vi "FeedbackDecode.vi"() -> ()   [LabVIEW 2020] (continued)
        n285 = call "FeedbackDecode_PlotHeatmap.vi"("Range"=w3314, "GridIntensity"=w3326, "Instance"=0, "Mode"=w3331) -> ("Pic"=w3317:picture)  [unwired: 2 in, 1 out]
        n286 = call "FeedbackDecode_PlotHeatmap.vi"("Range"=w3314, "GridIntensity"=w3325, "Instance"=1, "Mode"=w3331) -> ("Pic"=w3316:picture)  [unwired: 2 in, 1 out]
        n287 = call "FeedbackDecode_PlotHeatmap.vi"("Range"=w3314, "GridIntensity"=w3318, "Instance"=2, "Mode"=w3331) -> ("Pic"=w3315:picture)  [unwired: 2 in, 1 out]
        n288 = local write "MedianHM"(w3317) -> ()
        n289 = local write "UlnarHM"(w3316) -> ()
        n290 = local write "EMGHM"(w3315) -> ()
        n291 = for {
          tunnel: w3258 -> [w3411] mode=indexing
          tunnel: [w3410] -> w3260 mode=indexing
          tunnel: w3259 -> [w3407]
          tunnel: w3257 -> [w3409] mode=indexing
          tunnel: [w3406] -> w3256 mode=indexing
          n292 = Build Array(w3411) -> (w3412:dbl[])
          n293 = Build Array(w3409) -> (w3408:dbl[])
          n294 = Bundle By Name("Y"=w3412, "t0"=w3407) -> (w3410:waveform(dbl))  [unwired: 1 in]
          n295 = Bundle By Name("Y"=w3408, "t0"=w3407) -> (w3406:waveform(dbl))  [unwired: 1 in]
        }
        "TASKA Pressure" <- w3260
        "TASKA IR" <- w3256
        n296 = global read "FeedbackDecode_Globals.vi" "FD_PupilClust"() -> (→"PupilClust":T11)
        n297 = case shown="True" w3263 {
          frame False {
          }
          frame True {
            n298 = call <vilib>:"Play Sound File.vi"("path"=path "C:/Windows/Media/Windows Critical Stop.wav") -> ()  [unwired: 9 in, 2 out]
          }
        }
        n299 = local read "CurrMvnt"() -> (w3397:T1)
        n300 = local read "MSMSSphere"() -> (w3350:dbl[][])
        n301 = local read "BaseCnt3"() -> (w3266:i64)
        n302 = local read "LoopCnt"() -> (w3290:u64)
        n303 = case shown="\"Training\"" w3287 {
          tunnel: w3311 -> [_ _ w3492]
          tunnel: [T26 {"[0]"=0.0, "[1]"=0.0, "[2]"=0.0, "[3]"=0.0, "[4]"=0.0, "[5]"=0.0, "[6]"=0.0, "[7]"=0.0, "[8]"=0.0, "[9]"=0.0, "[10]"=0.0, "[11]"=0.0} ("Kinematics") w3491 w3492] -> w3346
          tunnel: w3312 -> [_ w3491 _]
          frame "Off" {
          }
          frame "Training" {
          }
          frame "Decode", Default {
          }
        }
        n304 = local read "MSMSMvnt"() -> (w3351:dbl[])
        n305 = Unbundle By Name(w3397) -> ("Radius"=w3252:dbl)
        n306 = Equal?(x=w3290, y=w3266) -> (x = y?=w3291:bool)
        n307 = Replace Array Subset(array=w3350, new element=w3392, index (row)=0 ("disabled index (row)"), index (col)=0 ("disabled index (col)")) -> (w3254:dbl[][])
        n308 = Cluster To Array(cluster=w3346) -> (array=w3310:dbl[])
        n309 = case shown="True" w3291 {
          frame False {
          }
          frame True {
            n310 = local read "PulseStim"() -> (w3435:bool)
            n311 = case shown="True" w3435 {
              frame False {
                n312 = local read "EncodeClust"() -> (w3438:T9)
                n313 = local write "PulseStim"(TRUE ("PulseStim")) -> ()
                n314 = local read "EncodeClust"() -> (w3442:T9)
                n315 = Unbundle By Name(w3438) -> ("Wait Period"=w3439:dbl)
                n316 = Unbundle By Name(w3442) -> ("Pulse"=w3441:bool)
                n317 = local read "LoopCnt"() -> (w3437:u64)
                n318 = expression code="x*100"(w3439) -> (w3440:dbl)
                n319 = case shown="True" w3441 {
                  tunnel: ["SS.PulseStim=1;" ("EventStr") "SS.PulseStim=0;" ("EventStr")] -> w3444
                  frame False {
                  }
                  frame True {
                  }
                }
                n320 = Add(x=w3437, y=w3440) -> (x+y=w3436:dbl)
                n321 = local write "BaseCnt3"(w3436) -> ()
                n322 = local read "DecodeClust"() -> (w3445:T5)
                n323 = Bundle By Name(cluster=w3445, "EventStr"=w3444) -> (w3447:T5)
                n324 = call "FeedbackDecode_MLComCtrl.vi"("DecodeClustIn"=w3447, "Mode"=T19."SendEvent") -> ()  [unwired: 6 in, 4 out]
              }
              frame True {
                n325 = local read "EncodeClust"() -> (w3452:T9)
                n326 = local write "PulseStim"(FALSE ("PulseStim")) -> ()
                n327 = Unbundle By Name(w3452) -> ("Train Period"=w3453:dbl)
                n328 = local read "LoopCnt"() -> (w3451:u64)
                n329 = expression code="x*100"(w3453) -> (w3454:dbl)
                n330 = Add(x=w3451, y=w3454) -> (x+y=w3450:dbl)
                n331 = local read "DecodeClust"() -> (w3457:T5)
                n332 = local write "BaseCnt3"(w3450) -> ()
                n333 = Bundle By Name(cluster=w3457, "EventStr"="SS.PulseStim=1;") -> (w3459:T5)
                n334 = call "FeedbackDecode_MLComCtrl.vi"("DecodeClustIn"=w3459, "Mode"=T19."SendEvent") -> ()  [unwired: 6 in, 4 out]
              }
            }
          }
        }
        n335 = In Range and Coerce(upper limit=1.0, x=w3310, lower limit=-1.0) -> (coerced(x)=w3353:dbl[])  [unwired: 1 out]
        n336 = Unbundle By Name(w3295) -> ("CtrlButtons.HideSphrs"=w3298:bool)
        n337 = Initialize Array(w3252, 6 ("dimension size")) -> (w3250:dbl[])
        n338 = call "FeedbackDecode_InWindowMDim.vi"("Radius"=w3252, "Targ"=w3302, "Pos"=w3353) -> ("Status"=w3345:enum16{"In", "Out"}, "TargStatus"=w3349:i16[], "TargDist"=w3344:dbl[])  [unwired: 1 in, 1 out]
        n339 = case shown="\"Acquire Start\"" w3405 {
          tunnel: w3345 -> [_ w3591 w3668 _]
          frame "Initialize", Default {
            n340 = local read "DecodeClust"() -> (w3503:T5)
            n341 = Unbundle By Name(w3503) -> ("TestType"=w3501:T23, "CtrlButtons.StartTrials"=w3498:bool, "KinSrc"=w3502:T37)
            n342 = Equal?(x=T30."MSMS", y=w3501) -> (x = y?=w3499:bool)
            n343 = And(x=w3499, y=w3498) -> (x .and. y?=w3497:bool)
            n344 = case shown="True" w3497 {
              tunnel: w3502 -> [_ w3504]
              frame False {
              }
              frame True {
                n345 = stacked-sequence {
                  tunnel: w3504 -> [w3511 _]
                  frame #0 {
                    w3513 = enum16{"Initialize", "Reset", "Run"}."Initialize" ("Mode")
                    # "For step targets, the duration of step is set to ART+ARTR and ARD/ETD are a function of the hold and rise times of the movement."
                    n346 = local read "MvntBuilder"() -> (w3508:T6)
                    n347 = Unbundle By Name(w3508) -> ("MvntList"=w3526:T24)
                    n348 = Unbundle By Name(w3508) -> ("TargParams.Gain"=w3515:dbl, "TargParams.Acc"=w3531:dbl, "Mode"=w3527:enum16{"Selected", "Block", "Random"}, "NTrials"=w3529:dbl)
                    n349 = local read "Timing"() -> (w3535:T3)
                    n350 = Array Size(array=w3526) -> (size(s)=w3528:i32)
                    n351 = case shown="\"Block\", Default" w3527 {
                      selector: w3527 -> [_ w3541]
                      tunnel: [w3540 w3545] -> w3509
                      tunnel: w3528 -> [_ w3544]
                      tunnel: w3529 -> [_ w3543]
                      tunnel: [0.0 ("Perc") w3542] -> w3507
                      frame "Selected" {
                        n352 = property on="MvntList" class="Arr (strict)"() -> ("Index Values"=w3539:u32[])  [unwired: 2 in, 2 out]
                        n353 = Index Array(array=w3539) -> (element=w3540:u32)  [unwired: 1 in]
                      }
                      frame "Block", Default {
                        n354 = call "FeedbackDecode_GenRandBlockIdxs2.vi"("Mode"=w3541, "NumTrials"=w3543, "NumIdxs"=w3544) -> ("RandIdx"=w3545:dbl, "Perc"=w3542:dbl)  [unwired: 2 in]
                      }
                    }
                    "NextIdx" <- w3509
                    n355 = local read "LoopPeriod"() -> (w3514:u64)
                    n356 = Unbundle By Name(w3535) -> ("Dur.ART"=w3517:dbl, "Rnd.ARTR"=w3516:dbl)
                    n357 = Index Array(array=w3526, index=w3509) -> (element=w3505:T1)
                    n358 = Bundle By Name(cluster=w3508, "PercTrials"=w3507) -> (w3506:T6)
                    n359 = Unbundle By Name(w3505) -> ("Tracking"=w3520:enum8{"False", "True", "Mixed"})
                    n360 = Add(x=w3517, y=w3516) -> (x+y=w3518:dbl)
                    n361 = local write "CurrMvnt"(w3505) -> ()
                    n362 = Subtract(x=1.0, y=w3531) -> (x-y=w3533:dbl)
                    n363 = call "FeedbackDecode_GenContTarget.vi"("Gain"=w3515, "StepTime (ms)"=w3518, "MvntClust"=w3505, "LoopPeriod (ms)"=w3514, "Mode"=w3513) -> ()  [unwired: 1 in, 4 out]
                    n364 = call "FeedbackDecode_GenContMvnt.vi"("Mode"=w3513, "LoopPeriod"=w3514, "Gain"=w3515, "MvntClust"=w3505) -> ("MaxTimes (ms)"=w3519:T42)  [unwired: 2 in, 2 out]
                    n365 = local read "MvntEvnt"() -> (w3510:refnum<user-event>)
                    n366 = Unbundle By Name(w3519) -> ("Hold"=w3521:dbl, "Rise"=w3525:dbl, "Trial"=w3532:dbl)
                    n367 = Not Equal To 0?(x=w3520) -> (x != 0?=w3522:bool)
                    "Tracking" <- w3522
                    n368 = local write "MvntBuilder"(w3506) -> ()
                    n369 = Generate User Event(user event=w3510, event data cluster=w3509) -> ()  [unwired: 2 in, 2 out]
                    n370 = expression code="2*x"(w3525) -> (w3524:dbl)
                    n371 = Multiply(x=w3532, y=w3533) -> (x*y=w3534:dbl)
                    n372 = case shown="False" w3522 {
                      tunnel: w3535 -> [w3552 w3565]
                      tunnel: [w3551 w3564] -> w3512
                      tunnel: w3521 -> [w3550 _]
                      tunnel: w3524 -> [w3549 _]
                      tunnel: [w3546 w3562] -> w3523
                      tunnel: w3532 -> [w3547 w3562]
                      tunnel: w3511 -> [w3548 _]
                      tunnel: w3534 -> [_ w3561]
                      frame False {
                        n373 = case shown="\"Training\"" w3548 {
                          tunnel: w3552 -> [w3554 w3560]
                          tunnel: [w3554 w3559] -> w3551
                          tunnel: w3550 -> [_ w3558]
                          tunnel: w3549 -> [_ w3557]
                          tunnel: w3547 -> [w3553 w3556]
                          tunnel: [w3553 w3556] -> w3546
                          frame "Off", Default {
                          }
                          frame "Training" {
                            w3555 = u16 0 ("Rnd.ARDR")
                            n374 = Bundle By Name(cluster=w3560, "Rnd.ARDR"=w3555, "Dur.ARD"=w3558, "Dur.ETD"=w3557, "Rnd.ETDR"=w3555) -> (w3559:T3)
                          }
                        }
                      }
                      frame True {
                        n375 = Bundle By Name(cluster=w3565, "Rnd.ARTR"=u16 0, "Dur.ART"=w3562, "Dur.ETD"=w3561) -> (w3564:T3)
                      }
                    }
                    "TrialTime (ms)" <- w3523
                    n376 = local read "PrevIdx"() -> (w3536:dbl)
                    n377 = Not Equal?(x=w3509, y=w3536) -> (x != y?=w3537:bool)
                    n378 = case shown="True" w3537 {
                      tunnel: w3511 -> [_ w3570]
                      tunnel: w3512 -> [w3566 w3569]
                      frame False {
                        n379 = local write "iTiming"(w3566) -> ()
                      }
                      frame True {
                        n380 = case shown="\"Training\"" w3570 {
                          tunnel: w3569 -> [w3571 w3572]
                          frame "Off", Default {
                            n381 = local write "iTiming"(w3571) -> ()
                          }
                          frame "Training" {
                            n382 = Unbundle By Name(w3572) -> ("Dur.ASD"=w3575:dbl)
                            n383 = Multiply(x=w3575, y=u16 2) -> (x*y=w3576:dbl)
                            n384 = Bundle By Name(cluster=w3572, "Dur.ASD"=w3576) -> (w3573:T3)
                            n385 = local write "iTiming"(w3573) -> ()
                          }
                        }
                        n386 = local read "LoopCnt"() -> (w3567:u64)
                        n387 = local write "ResetCorr"(TRUE ("ResetCorr")) -> ()
                        n388 = local write "BaseCnt1"(w3567) -> ()
                      }
                    }
                  }
                  frame #1 {
                    n389 = local write "Outcome"(enum16{"---", "Success", "Failure"}."---" ("Outcome")) -> ()
                    n390 = local read "NextIdx"() -> (w3577:dbl)
                    n391 = local read "LoopCnt"() -> (w3587:u64)
                    n392 = call "FeedbackDecode_RunOnce.vi"("Instance"=0, "Mode"=enum16{"Reset", "Run"}."Reset") -> ()  [unwired: 1 out]
                    n393 = local write "PrevIdx"(w3577) -> ()
                    n394 = call "FeedbackDecode_LoopComp.vi"("LoopCount"=w3587, "Instance"=0, "Mode"=enum16{"Reset", "Run"}."Reset") -> ()  [unwired: 3 in, 2 out]
                    n395 = call "FeedbackDecode_RunOnce.vi"("Instance"=1, "Mode"=enum16{"Reset", "Run"}."Reset") -> ()  [unwired: 1 out]
                    n396 = local write "State"(T16."Acquire Start" ("Current State")) -> ()
                    "TargCnt" <- u64 0 ("TargAcc")
                    "SubCase" <- 0 ("SubCase")
                  }
                }
              }
            }
          }
          frame "Acquire Start" {
            n397 = local read "iTiming"() -> (w3594:T3)
            n398 = Unbundle By Name(w3594) -> ("Dur.ASD"=w3589:dbl, "Rnd.ASDR"=w3593:dbl)
            n399 = Equal To 0?(x=w3589) -> (x = 0?=w3590:bool)
            n400 = case shown="True" w3590 {
              tunnel: [w3595 enum16{"In", "Out"}."In" ("Status")] -> w3592
              tunnel: w3591 -> [w3595 _]
              frame False {
              }
              frame True {
              }
            }
            n401 = case shown="\"In\", Default" w3592 {
              tunnel: w3589 -> [w3598 _]
              tunnel: w3593 -> [w3597 _]
              frame "In", Default {
                n402 = local read "LoopPeriod"() -> (w3606:u64)
                n403 = local read "LoopCnt"() -> (w3603:u64)
                n404 = local read "Timing"() -> (w3599:T3)
                n405 = call "FeedbackDecode_LoopComp.vi"("RandTime"=w3597, "LoopPeriod"=w3606, "SetTime"=w3598, "LoopCount"=w3603, "Instance"=0, "Mode"=enum16{"Reset", "Run"}."Run") -> ("ActualTime"=w3601:u64, "Outcome"=w3600:enum16{"TimeIn", "TimeOut"})
                n406 = Bundle By Name(cluster=w3599, "Act.ASDA"=w3601) -> (w3602:T3)
                n407 = local write "Timing"(w3602) -> ()
                n408 = case shown="\"TimeOut\"" w3600 {
                  frame "TimeIn", Default {
                    n409 = local read "DecodeClust"() -> (w3608:T5)
                    n410 = Unbundle By Name(w3608) -> ("CtrlButtons.ResetTrial"=w3607:bool)
                    n411 = case shown="True" w3607 {
                      frame False {
                      }
                      frame True {
                        n412 = local read "LoopCnt"() -> (w3611:u64)
                        n413 = local write "State"(T16."Finalize" ("Current State")) -> ()
                        n414 = call "FeedbackDecode_RunOnce.vi"("Instance"=0, "Mode"=enum16{"Reset", "Run"}."Reset") -> ()  [unwired: 1 out]
                        n415 = call "FeedbackDecode_LoopComp.vi"("LoopCount"=w3611, "Instance"=0, "Mode"=enum16{"Reset", "Run"}."Reset") -> ()  [unwired: 3 in, 2 out]
                      }
                    }
                  }
                  frame "TimeOut" {
                    n416 = local read "SubCase"() -> (w3615:i32)
                    n417 = case shown="1, Default" w3615 {
                      frame 0 {
                        # "This subcase delays the execution by 1 loop iteration"
                        n418 = local read "DecodeClust"() -> (w3618:T5)
                        n419 = Unbundle By Name(w3618) -> ("CtrlButtons.CalDEKA"=w3617:bool)
                        n420 = local write "SubCase"(1 ("SubCase")) -> ()
                        n421 = case shown="True" w3617 {
                          frame False {
                          }
                          frame True {
                            n422 = property on="HideSphrs" class="Bool (strict)"("Val(Sgnl)"=TRUE ("Value (Signaling)")) -> ()  [unwired: 2 in, 2 out]
                          }
                        }
                      }
                      frame 1, Default {
                        n423 = local read "LoopCnt"() -> (w3638:u64)
                        n424 = local read "CurrMvnt"() -> (w3620:T1)
                        n425 = local read "LoopCnt"() -> (w3641:u64)
                        n426 = local read "NIPTime"() -> (w3628:dbl)
                        n427 = local read "LoopCnt"() -> (w3633:u64)
                        n428 = Unbundle By Name(w3620) -> ("Radius"=w3623:dbl)
                        n429 = call "FeedbackDecode_GenContMvnt.vi"("Mode"=enum16{"Initialize", "Reset", "Run"}."Reset", "LoopCount"=w3641) -> ()  [unwired: 4 in, 3 out]
                        n430 = call "FeedbackDecode_GenContTarget.vi"("LoopCount"=w3638, "Mode"=enum16{"Initialize", "Reset", "Run"}."Reset") -> ()  [unwired: 4 in, 4 out]
                        n431 = call-poly "FeedbackDecode_VariablesToString.vi"("Format"="%0.0f", "ValueIn"=w3628, "FieldName"="NIPTime" ("Key Word")) -> ("StringOut"=w3631:string)  [unwired: 4 in]
                        n432 = Format Into String(w3633) -> (resulting string=w3625:string)  [unwired: 3 in, 1 out]
                        n433 = Concatenate Strings("TargOn:SS.EventID=" ("string"), w3625) -> (w3630:string)
                        n434 = call-poly "FeedbackDecode_VariablesToString.vi"("ValueIn"=w3623, "FieldName"="TargRad" ("Key Word")) -> ("StringOut"=w3621:string)  [unwired: 5 in]
                        n435 = local read "LoopCnt"() -> (w3647:u64)
                        n436 = local read "EventParamsFID"() -> (w3627:refnum<file>)
                        n437 = Concatenate Strings(w3630, ";" ("string"), w3631, w3621) -> (w3624:string)
                        n438 = call "FeedbackDecode_WriteTextEOL.vi"("text"=w3624, "refnum in"=w3627) -> ()  [unwired: 8 in, 2 out]
                        n439 = call "FeedbackDecode_LoopComp.vi"("LoopCount"=w3647, "Instance"=0, "Mode"=enum16{"Reset", "Run"}."Reset") -> ()  [unwired: 3 in, 2 out]
                        n440 = local read "DecodeClust"() -> (w3637:T5)
                        n441 = Bundle By Name(cluster=w3637, "EventStr"=w3624) -> (w3635:T5)
                        n442 = local read "LoopCnt"() -> (w3644:u64)
                        n443 = call "FeedbackDecode_MLComCtrl.vi"("DecodeClustIn"=w3635, "Mode"=T19."SendEvent") -> ()  [unwired: 6 in, 4 out]
                        n444 = local write "State"(T16."Acquire Response" ("Current State")) -> ()
                        n445 = call "FeedbackDecode_LoopComp.vi"("LoopCount"=w3644, "Instance"=1, "Mode"=enum16{"Reset", "Run"}."Reset") -> ()  [unwired: 3 in, 2 out]
                      }
                    }
                  }
                }
              }
              frame "Out" {
                n446 = local read "LoopCnt"() -> (w3653:u64)
                n447 = call "FeedbackDecode_LoopComp.vi"("LoopCount"=w3653, "Instance"=0, "Mode"=enum16{"Reset", "Run"}."Reset") -> ()  [unwired: 3 in, 2 out]
                n448 = local read "DecodeClust"() -> (w3650:T5)
                n449 = Unbundle By Name(w3650) -> ("CtrlButtons.ResetTrial"=w3649:bool)
                n450 = case shown="True" w3649 {
                  frame False {
                  }
                  frame True {
                    n451 = call "FeedbackDecode_RunOnce.vi"("Instance"=0, "Mode"=enum16{"Reset", "Run"}."Reset") -> ()  [unwired: 1 out]
                    n452 = local write "State"(T16."Finalize" ("Current State")) -> ()
                  }
                }
              }
            }
          }
          frame "Acquire Response" {
            n453 = local read "Timing"() -> (w3657:T3)
            n454 = local read "iTiming"() -> (w3663:T3)
            n455 = local read "LoopPeriod"() -> (w3659:u64)
            n456 = local read "LoopCnt"() -> (w3662:u64)
            n457 = Unbundle By Name(w3663) -> ("Dur.ART"=w3665:dbl, "Rnd.ARTR"=w3666:dbl)
            n458 = call "FeedbackDecode_LoopComp.vi"("RandTime"=w3666, "LoopPeriod"=w3659, "SetTime"=w3665, "LoopCount"=w3662, "Instance"=1, "Mode"=enum16{"Reset", "Run"}."Run") -> ("ActualTime"=w3667:u64, "Outcome"=w3658:enum16{"TimeIn", "TimeOut"})
            n459 = Bundle By Name(cluster=w3657, "Act.ARTA"=w3667) -> (w3664:T3)
            n460 = local write "Timing"(w3664) -> ()
            n461 = case shown="\"TimeOut\"" w3658 {
              tunnel: w3668 -> [w3669 _]
              frame "TimeIn", Default {
                n462 = case shown="\"Out\"" w3669 {
                  frame "In", Default {
                    n463 = local read "Tracking"() -> (w3670:bool)
                    n464 = case shown="False" w3670 {
                      tunnel: [w3673 w3685] -> w3671
                      frame False {
                        n465 = local read "Timing"() -> (w3672:T3)
                        n466 = local read "iTiming"() -> (w3678:T3)
                        n467 = local read "LoopPeriod"() -> (w3682:u64)
                        n468 = local read "LoopCnt"() -> (w3679:u64)
                        n469 = Unbundle By Name(w3678) -> ("Dur.ARD"=w3676:dbl, "Rnd.ARDR"=w3675:dbl)
                        n470 = call "FeedbackDecode_LoopComp.vi"("RandTime"=w3675, "LoopPeriod"=w3682, "SetTime"=w3676, "LoopCount"=w3679, "Instance"=0, "Mode"=enum16{"Reset", "Run"}."Run") -> ("ActualTime"=w3674:u64, "Outcome"=w3673:enum16{"TimeIn", "TimeOut"})
                        n471 = Bundle By Name(cluster=w3672, "Act.ARDA"=w3674) -> (w3677:T3)
                        n472 = local write "Timing"(w3677) -> ()
                      }
                      frame True {
                        n473 = local read "TargCnt"() -> (w3686:u64)
                        n474 = local read "MvntBuilder"() -> (w3684:T6)
                        n475 = local read "TrialTime (ms)"() -> (w3690:dbl)
                        n476 = local read "LoopPeriod"() -> (w3688:u64)
                        n477 = Increment(x=w3686) -> (x+1=w3687:u64)
                        n478 = Unbundle By Name(w3684) -> ("TargParams.Acc"=w3683:dbl)
                        n479 = Multiply(x=w3687, y=w3688) -> (x*y=w3691:u64)
                        n480 = Multiply(x=w3690, y=w3683) -> (x*y=w3689:dbl)
                        n481 = local write "TargCnt"(w3687) -> ()
                        n482 = Greater Or Equal?(x=w3691, y=w3689) -> (x >= y?=w3692:bool)
                        n483 = Boolean To (0,1)(Boolean=w3692) -> (0, 1=w3685:i16)
                      }
                    }
                    n484 = case shown="0, Default" w3671 {
                      frame 0, Default {
                        # "TimeIn"
                        n485 = local read "DecodeClust"() -> (w3694:T5)
                        n486 = Unbundle By Name(w3694) -> ("CtrlButtons.ResetTrial"=w3693:bool)
                        n487 = call "FeedbackDecode_RunOnce.vi"("Instance"=0, "Mode"=enum16{"Reset", "Run"}."Run") -> ("State"=w3697:enum16{"RunOnce", "Finished"})
                        n488 = case shown="\"RunOnce\", Default" w3697 {
                          tunnel: w3693 -> [_ w3711]
                          frame "RunOnce", Default {
                            n489 = local read "NIPTime"() -> (w3703:dbl)
                            n490 = local read "LoopCnt"() -> (w3709:u64)
                            n491 = Format Into String(w3709) -> (resulting string=w3700:string)  [unwired: 3 in, 1 out]
                            n492 = call-poly "FeedbackDecode_VariablesToString.vi"("Format"="%0.0f", "ValueIn"=w3703, "FieldName"="NIPTime" ("Key Word")) -> ("StringOut"=w3706:string)  [unwired: 4 in]
                            n493 = local read "EventParamsFID"() -> (w3702:refnum<file>)
                            n494 = Concatenate Strings("InTarg:SS.EventID=" ("string"), w3700) -> (w3705:string)
                            n495 = Concatenate Strings(w3705, ";" ("string"), w3706) -> (w3707:string)
                            n496 = call "FeedbackDecode_WriteTextEOL.vi"("text"=w3707, "refnum in"=w3702) -> ()  [unwired: 8 in, 2 out]
                          }
                          frame "Finished" {
                            n497 = case shown="False" w3711 {
                              frame False {
                              }
                              frame True {
                                n498 = local read "LoopCnt"() -> (w3712:u64)
                                n499 = call "FeedbackDecode_LoopComp.vi"("LoopCount"=w3712, "Instance"=0, "Mode"=enum16{"Reset", "Run"}."Reset") -> ()  [unwired: 3 in, 2 out]
                                n500 = local write "State"(T16."Finalize" ("Current State")) -> ()
                                n501 = call "FeedbackDecode_RunOnce.vi"("Instance"=0, "Mode"=enum16{"Reset", "Run"}."Reset") -> ()  [unwired: 1 out]
                              }
                            }
                          }
                        }
                        n502 = call "FeedbackDecode_RunOnce.vi"("Instance"=1, "Mode"=enum16{"Reset", "Run"}."Reset") -> ()  [unwired: 1 out]
                      }
                      frame 1 {
                        # "TimeOut"
                        n503 = local read "LoopCnt"() -> (w3733:u64)
                        n504 = call "FeedbackDecode_LoopComp.vi"("LoopCount"=w3733, "Instance"=1, "Mode"=enum16{"Reset", "Run"}."Reset") -> ()  [unwired: 3 in, 2 out]
                        n505 = call "FeedbackDecode_RunOnce.vi"("Instance"=0, "Mode"=enum16{"Reset", "Run"}."Reset") -> ()  [unwired: 1 out]
                        n506 = local read "LoopCnt"() -> (w3740:u64)
                        n507 = call "FeedbackDecode_LoopComp.vi"("LoopCount"=w3740, "Instance"=0, "Mode"=enum16{"Reset", "Run"}."Reset") -> ()  [unwired: 3 in, 2 out]
                        n508 = local write "State"(T16."Finalize" ("Current State")) -> ()
                        n509 = local read "NIPTime"() -> (w3725:dbl)
                        n510 = local read "LoopCnt"() -> (w3730:u64)
                        n511 = local write "Outcome"(enum16{"---", "Success", "Failure"}."Success" ("Outcome")) -> ()
                        n512 = Format Into String(w3730) -> (resulting string=w3722:string)  [unwired: 3 in, 1 out]
                        n513 = call-poly "FeedbackDecode_VariablesToString.vi"("Format"="%0.0f", "ValueIn"=w3725, "FieldName"="NIPTime" ("Key Word")) -> ("StringOut"=w3728:string)  [unwired: 4 in]
                        n514 = local read "EventParamsFID"() -> (w3724:refnum<file>)
                        n515 = Concatenate Strings("Success:SS.EventID=" ("string"), w3722) -> (w3727:string)
                        n516 = Concatenate Strings(w3727, ";" ("string"), w3728) -> (w3718:string)
                        n517 = call "FeedbackDecode_WriteTextEOL.vi"("text"=w3718, "refnum in"=w3724) -> ()  [unwired: 8 in, 2 out]
                        n518 = local read "DecodeClust"() -> (w3721:T5)
                        n519 = Bundle By Name(cluster=w3721, "EventStr"=w3718) -> (w3719:T5)
                        n520 = call "FeedbackDecode_MLComCtrl.vi"("DecodeClustIn"=w3719, "Mode"=T19."SendEvent") -> ()  [unwired: 6 in, 4 out]
                      }
                    }
                  }
                  frame "Out" {
                    n521 = local read "DecodeClust"() -> (w3743:T5)
                    n522 = Unbundle By Name(w3743) -> ("CtrlButtons.ResetTrial"=w3742:bool)
                    n523 = case shown="True" w3742 {
                      frame False {
                      }
                      frame True {
                        n524 = local write "State"(T16."Finalize" ("Current State")) -> ()
                      }
                    }
                    n525 = local read "LoopCnt"() -> (w3751:u64)
                    n526 = call "FeedbackDecode_LoopComp.vi"("LoopCount"=w3751, "Instance"=0, "Mode"=enum16{"Reset", "Run"}."Reset") -> ()  [unwired: 3 in, 2 out]
                    n527 = call "FeedbackDecode_RunOnce.vi"("Instance"=1, "Mode"=enum16{"Reset", "Run"}."Run") -> ("State"=w3746:enum16{"RunOnce", "Finished"})
                    n528 = call "FeedbackDecode_RunOnce.vi"("Instance"=0, "Mode"=enum16{"Reset", "Run"}."Reset") -> ()  [unwired: 1 out]
                    n529 = case shown="\"RunOnce\", Default" w3746 {
                      frame "RunOnce", Default {
                        n530 = local read "NIPTime"() -> (w3755:dbl)
                        n531 = local read "LoopCnt"() -> (w3761:u64)
                        n532 = Format Into String(w3761) -> (resulting string=w3752:string)  [unwired: 3 in, 1 out]
                        n533 = call-poly "FeedbackDecode_VariablesToString.vi"("Format"="%0.0f", "ValueIn"=w3755, "FieldName"="NIPTime" ("Key Word")) -> ("StringOut"=w3758:string)  [unwired: 4 in]
                        n534 = local read "EventParamsFID"() -> (w3754:refnum<file>)
                        n535 = Concatenate Strings("OutTarg:SS.EventID=" ("string"), w3752) -> (w3757:string)
                        n536 = Concatenate Strings(w3757, ";" ("string"), w3758) -> (w3759:string)
                        n537 = call "FeedbackDecode_WriteTextEOL.vi"("text"=w3759, "refnum in"=w3754) -> ()  [unwired: 8 in, 2 out]
                      }
                      frame "Finished" {
                      }
                    }
                  }
                }
              }
              frame "TimeOut" {
                n538 = local read "LoopCnt"() -> (w3786:u64)
                n539 = local read "LoopCnt"() -> (w3779:u64)
                n540 = call "FeedbackDecode_RunOnce.vi"("Instance"=0, "Mode"=enum16{"Reset", "Run"}."Reset") -> ()  [unwired: 1 out]
                n541 = call "FeedbackDecode_LoopComp.vi"("LoopCount"=w3786, "Instance"=0, "Mode"=enum16{"Reset", "Run"}."Reset") -> ()  [unwired: 3 in, 2 out]
                n542 = call "FeedbackDecode_LoopComp.vi"("LoopCount"=w3779, "Instance"=1, "Mode"=enum16{"Reset", "Run"}."Reset") -> ()  [unwired: 3 in, 2 out]
                n543 = local write "Outcome"(enum16{"---", "Success", "Failure"}."Failure" ("Outcome")) -> ()
                n544 = local write "State"(T16."Finalize" ("Current State")) -> ()
                n545 = local read "NIPTime"() -> (w3771:dbl)
                n546 = local read "LoopCnt"() -> (w3776:u64)
                n547 = Format Into String(w3776) -> (resulting string=w3768:string)  [unwired: 3 in, 1 out]
                n548 = call-poly "FeedbackDecode_VariablesToString.vi"("Format"="%0.0f", "ValueIn"=w3771, "FieldName"="NIPTime" ("Key Word")) -> ("StringOut"=w3774:string)  [unwired: 4 in]
                n549 = local read "EventParamsFID"() -> (w3770:refnum<file>)
                n550 = Concatenate Strings("Failure:SS.EventID=" ("string"), w3768) -> (w3773:string)
                n551 = Concatenate Strings(w3773, ";" ("string"), w3774) -> (w3764:string)
                n552 = call "FeedbackDecode_WriteTextEOL.vi"("text"=w3764, "refnum in"=w3770) -> ()  [unwired: 8 in, 2 out]
                n553 = local read "DecodeClust"() -> (w3767:T5)
                n554 = Bundle By Name(cluster=w3767, "EventStr"=w3764) -> (w3765:T5)
                n555 = call "FeedbackDecode_MLComCtrl.vi"("DecodeClustIn"=w3765, "Mode"=T19."SendEvent") -> ()  [unwired: 6 in, 4 out]
              }
            }
          }
          frame "Finalize" {
            # "End of trial delay"
            n556 = local read "Timing"() -> (w3788:T3)
            n557 = local read "iTiming"() -> (w3792:T3)
            n558 = local read "LoopPeriod"() -> (w3795:u64)
            n559 = local read "LoopCnt"() -> (w3798:u64)
            n560 = Unbundle By Name(w3792) -> ("Dur.ETD"=w3791:dbl, "Rnd.ETDR"=w3790:dbl)
            n561 = call "FeedbackDecode_LoopComp.vi"("RandTime"=w3790, "LoopPeriod"=w3795, "SetTime"=w3791, "LoopCount"=w3798, "Instance"=0, "Mode"=enum16{"Reset", "Run"}."Run") -> ("ActualTime"=w3789:u64, "Outcome"=w3794:enum16{"TimeIn", "TimeOut"})
            n562 = Bundle By Name(cluster=w3788, "Act.ETDA"=w3789) -> (w3793:T3)
            n563 = local write "Timing"(w3793) -> ()
            n564 = case shown="\"TimeOut\"" w3794 {
              frame "TimeIn", Default {
                n565 = call "FeedbackDecode_RunOnce.vi"("Instance"=0, "Mode"=enum16{"Reset", "Run"}."Run") -> ("State"=w3799:enum16{"RunOnce", "Finished"})
                n566 = case shown="\"RunOnce\", Default" w3799 {
                  frame "RunOnce", Default {
                    n567 = local read "DecodeClust"() -> (w3805:T5)
                    n568 = Unbundle By Name(w3805) -> ("CtrlButtons.CalDEKA"=w3804:bool)
                    n569 = case shown="True" w3804 {
                      frame False {
                      }
                      frame True {
                        n570 = property on="HideSphrs" class="Bool (strict)"("Val(Sgnl)"=FALSE ("Value (Signaling)")) -> ()  [unwired: 2 in, 2 out]
                      }
                    }
                    n571 = call "FeedbackDecode_GenContTarget.vi"("LoopCount"=-inf, "Mode"=enum16{"Initialize", "Reset", "Run"}."Reset") -> ()  [unwired: 4 in, 4 out]
                    n572 = local read "Outcome"() -> (w3806:enum16{"---", "Success", "Failure"})
                    n573 = case shown="\"Failure\"" w3806 {
                      frame "---", Default {
                      }
                      frame "Success" {
                        n574 = local read "PSRef"() -> (w3811:refnum<vi>)
                        n575 = call-by-ref "Start Asynchronous Call"(reference=w3811, "Mode"=enum16{"Cue", "Success", "Failure", "Abort"}."Success", "#S"=1000.0, "Fs"=5000.0) -> ()  [unwired: 10 in, 2 out]
                      }
                      frame "Failure" {
                        n576 = local read "PSRef"() -> (w3815:refnum<vi>)
                        n577 = call-by-ref "Start Asynchronous Call"(reference=w3815, "Mode"=enum16{"Cue", "Success", "Failure", "Abort"}."Failure", "#S"=1000.0 ("Volume"), "Fs"=5000.0) -> ()  [unwired: 10 in, 2 out]
                      }
                    }
                  }
                  frame "Finished" {
                  }
                }
              }
              frame "TimeOut" {
                n578 = local read "DecodeClust"() -> (w3825:T5)
                n579 = local read "MvntBuilder"() -> (w3816:T6)
                n580 = local read "CurrMvnt"() -> (w3823:T1)
                n581 = local read "Outcome"() -> (w3827:enum16{"---", "Success", "Failure"})
                n582 = call "FeedbackDecode_UpdateTrialCnt.vi"("DecodeClustIn"=w3825, "CurrMvnt"=w3823) -> ("DecodeClustOut"=w3824:T5)  [unwired: 1 in]
                n583 = Bundle By Name(cluster=w3824, "Outcome"=w3827) -> (w3826:T5)
                n584 = local read "Timing"() -> (w3840:T3)
                n585 = Unbundle By Name(w3816) -> ("TargParams"=w3841:cluster{"Gain":dbl, "Radius":dbl, "Acc":dbl})
                n586 = local read "EncodeClust"() -> (w3830:T9)
                n587 = local read "TrialArray"() -> (w3839:string[])
                n588 = local read "LoopCnt"() -> (w3821:u64)
                n589 = local read "NIPTime"() -> (w3822:dbl)
                n590 = call "FeedbackDecode_FPPNS2NIP.vi"("NIPTime"=w3822, "EncodeClust"=w3830, "LoopCnt"=w3821, "DecodeClust"=w3826, "TrialTiming"=w3840, "TargParams"=w3841, "MvntClust"=w3823) -> ("TrialParams"=w3832:string)  [unwired: 4 in]
                n591 = Match Pattern(string=w3832, regular expression="SS.MvntMat=\\[[-0-9,;\\.]+\\];") -> (match substring=w3837:string)  [unwired: 1 in, 3 out]
                n592 = local read "EventParamsFID"() -> (w3831:refnum<file>)
                n593 = Insert Into Array(array=w3839, new element=w3832) -> (w3838:string[])  [unwired: 1 in]
                n594 = Concatenate Strings("EndTrial:" ("String"), w3837) -> (w3833:string)
                n595 = Bundle By Name(cluster=w3826, "EventStr"=w3833) -> (w3829:T5)
                n596 = local write "TrialArray"(w3838) -> ()
                n597 = Unbundle By Name(w3816) -> ("PercTrials"=w3817:dbl)
                n598 = call "FeedbackDecode_WriteTextEOL.vi"("text"=w3832, "refnum in"=w3831) -> ()  [unwired: 8 in, 2 out]
                n599 = call "FeedbackDecode_MLComCtrl.vi"("DecodeClustIn"=w3829, "Mode"=T19."SendEvent") -> ("DecodeClustOut"=w3828:T5)  [unwired: 6 in, 3 out]
                n600 = Equal?(x=w3817, y=1.0) -> (x = y?=w3818:bool)
                n601 = Unbundle By Name(w3828) -> ("CtrlButtons.ResetTrial"=w3820:bool)
                n602 = case shown="False" w3820 {
                  tunnel: w3828 -> [w3844 w3879]
                  tunnel: w3818 -> [w3845 _]
                  tunnel: w3816 -> [w3843 _]
                  frame False {
                    n603 = case shown="True" w3845 {
                      tunnel: w3843 -> [_ w3850]
                      tunnel: w3844 -> [w3846 w3849]
                      frame False {
                        n604 = local write "DecodeClust"(w3846) -> ()
                      }
                      frame True {
                        n605 = flat-sequence {
                          tunnel: w3850 -> [w3853]
                          tunnel: w3849 -> [w3856]
                          tunnel: [w3855] -> w3848
                          tunnel: [w3854] -> w3847
                          tunnel: w3848 -> [w3866]
                          tunnel: w3847 -> [w3865]
                          frame #0 {
                            n606 = Unbundle By Name(w3853) -> ("Mode"=w3862:enum16{"Selected", "Block", "Random"}, "NTrials"=w3860:dbl, "MvntList"=w3859:T24)
                            n607 = local write "DecodeClust"(w3856) -> ()
                            n608 = Unbundle By Name(w3856) -> ("CtrlButtons.AcqTraining"=w3855:bool, "CtrlButtons.StartTrials"=w3854:bool)
                            n609 = Array Size(array=w3859) -> (size(s)=w3858:i32)
                            n610 = call "FeedbackDecode_GenRandBlockIdxs2.vi"("Mode"=w3862, "Reset"=TRUE, "NumTrials"=w3860, "NumIdxs"=w3858, "CurrIdx"=0.0) -> ("Perc"=w3852:dbl)  [unwired: 1 out]
                            n611 = Bundle By Name(cluster=w3853, "PercTrials"=w3852) -> (w3851:T6)
                            n612 = local write "MvntBuilder"(w3851) -> ()
                          }
                          frame #1 {
                            n613 = Build Array(w3866, w3865) -> (w3864:bool[])
                            n614 = Boolean Array To Number(Boolean array=w3864) -> (number=w3863:u32)
                            n615 = case shown="3" w3863 {
                              frame 0, Default {
                              }
                              frame 1 {
                                n616 = local read "MvntEvnt"() -> (w3867:refnum<user-event>)
                                n617 = property on="AcqTraining" class="Bool (strict)"("Val(Sgnl)"=FALSE ("Value (Signaling)")) -> ()  [unwired: 2 in, 2 out]
                                n618 = Generate User Event(user event=w3867, event data cluster=0.0 ("event data")) -> ()  [unwired: 2 in, 2 out]
                              }
                              frame 2 {
                                n619 = local read "MvntEvnt"() -> (w3870:refnum<user-event>)
                                n620 = property on="StartTrials" class="Bool (strict)"("Val(Sgnl)"=FALSE ("Value (Signaling)")) -> ()  [unwired: 2 in, 2 out]
                                n621 = Generate User Event(user event=w3870, event data cluster=0.0 ("event data")) -> ()  [unwired: 2 in, 2 out]
                              }
                              frame 3 {
                                w3876 = FALSE ("Value (Signaling)")
                                n622 = local read "MvntEvnt"() -> (w3873:refnum<user-event>)
                                n623 = property on="StartTrials" class="Bool (strict)"("Value"=w3876) -> (error out=w3875:errorcluster)  [unwired: 2 in, 1 out]
                                n624 = property on="AcqTraining" class="Bool (strict)"(error in=w3875, "Val(Sgnl)"=w3876) -> ()  [unwired: 1 in, 2 out]
                                n625 = Generate User Event(user event=w3873, event data cluster=0.0 ("event data")) -> ()  [unwired: 2 in, 2 out]
                              }
                            }
                          }
                        }
                      }
                    }
                  }
                  frame True {
                    n626 = Bundle By Name(cluster=w3879, "CtrlButtons.ResetTrial"=FALSE) -> (w3877:T5)
                    n627 = local write "DecodeClust"(w3877) -> ()
                  }
                }
                n628 = local write "State"(T16."Initialize" ("Current State")) -> ()
              }
            }
          }
        }
        n629 = Replace Array Subset(array=w3351, new element=w3353) -> (w3286:dbl[])  [unwired: 1 in]
        n630 = Replace Array Subset(array=w3254, new element=w3250, index (col)=3 ("disabled index (col)")) -> (w3253:dbl[][])  [unwired: 1 in]
        n631 = Replace Array Subset(array=w3253, new element=w3349, index (col)=4 ("disabled index (col)")) -> (w3300:dbl[][])  [unwired: 1 in]
        n632 = local write "Status"(w3345) -> ()
        n633 = local write "MSMSMvnt"(w3286) -> ()
        n634 = local write "TargDist"(w3344) -> ()
        n635 = case shown="True" w3298 {
          tunnel: w3300 -> [w3461 w3465]
          tunnel: [w3460 w3464] -> w3299
          frame False {
            n636 = Replace Array Subset(array=w3461, new element=dbl[] [1.0, 1.0, 1.0, 1.0, 1.0, 1.0] ("new element/subarray"), index (col)=5 ("disabled index (col)")) -> (w3460:dbl[][])  [unwired: 1 in]
          }
          frame True {
            n637 = Replace Array Subset(array=w3465, new element=dbl[] [0.0, 0.0, 0.0, 0.0, 0.0, 0.0] ("new element/subarray"), index (col)=5 ("disabled index (col)")) -> (w3464:dbl[][])  [unwired: 1 in]
          }
        }
        n638 = Unbundle By Name(w3289) -> ("CtrlButtons.ConnDEKA"=w3288:bool, "KMvntClust.CtrlMode"=w3285:T43, "KMvntClust.CtrlSpd"=w3281:sgl[], "KinSrc"=w3279:T37, "DEKAMode"=w3275:enum16{"Velocity", "Position"}, "CtrlButtons.CalDEKA"=w3282:bool)
        n639 = global write "FeedbackDecode_Globals.vi" "FD_MSMSMvnt"(w3286) -> ()
        n640 = call "FeedbackDecode_CombineMSMSPackets.vi"("SphereArray"=w3299, "MvntArray"=w3286) -> ()  [unwired: 1 in]
        n641 = local write "MSMSSphere"(w3299) -> ()
        n642 = case shown="False" w3282 {
          tunnel: w3282 -> [_ w3430]
          frame False {
          }
          frame True {
            n643 = call "FeedbackDecode_RunOnce.vi"("Instance"=2, "Mode"=enum16{"Reset", "Run"}."Run") -> ("State"=w3431:enum16{"RunOnce", "Finished"})
            n644 = case shown="\"RunOnce\", Default" w3431 {
              tunnel: w3430 -> [w3434 _]
              frame "RunOnce", Default {
                n645 = global write "FeedbackDecode_Globals.vi" "FD_CalDEKA"(w3434) -> ()
              }
              frame "Finished" {
              }
            }
          }
        }
        n646 = global write "FeedbackDecode_Globals.vi" "FD_ConnDEKA"(w3288) -> ()
        n647 = global write "FeedbackDecode_Globals.vi" "FD_CtrlMode"(w3285) -> ()
        n648 = global write "FeedbackDecode_Globals.vi" "FD_CtrlSpeed"(w3281) -> ()
        n649 = global write "FeedbackDecode_Globals.vi" "FD_KinSrc"(w3279) -> ()
        n650 = global write "FeedbackDecode_Globals.vi" "FD_DEKAMode"(w3275) -> ()
        n651 = global read "FeedbackDecode_Globals.vi" "FD_Stop"() -> (w3280:bool)
        n652 = node-c288() -> ()  [unwired: 1 in, 1 out]
        "LoopCnt" <- w3398
      }
      n653 = control-ref of="RespStr"() -> (w328:refnum<vi>)
      n654 = call "FeedbackDecode_PickROI.vi"("RespStrRef"=w328) -> ()  [unwired: 3 in]
      n655 = call "FeedbackDecode_PickROI_Adv.vi"("RespStrRef"=w328) -> ()  [unwired: 3 in]
      n656 = local read "PupilTracker"() -> (w327:bool)
      n657 = while {
        stop <- w338 stop-if-true
        n658 = Wait (ms)(milliseconds to wait=u32 1000) -> ()  [unwired: 1 out]
        n659 = local read "DataPath"() -> (w337:path)
        n660 = global read "FeedbackDecode_Globals.vi" "FD_Stop"() -> (w338:bool)
        n661 = call "FeedbackDecode_RecordAV.vi"("FullDataPath"=w337) -> ()  [unwired: 3 in]
      }
      n662 = case shown="True" w327 {
        frame False {
        }
        frame True {
          n663 = while {
            stop <- w332 stop-if-true
            n664 = local read "DataPath"() -> (w331:path)
            n665 = Wait (ms)(milliseconds to wait=u32 1000) -> ()  [unwired: 1 out]
            n666 = global read "FeedbackDecode_Globals.vi" "FD_Stop"() -> (w332:bool)
            n667 = call "FeedbackDecode_GetPupilInfo.vi"("FullDataPath"=w331) -> ()  [unwired: 3 in]
          }
        }
      }
      n668 = while {
        stop <- w341 stop-if-true
        n669 = local read "EvntReg"() -> (w340:refnum<event-registration>)
        n670 = event shown="[92] \"EncodeClust.ManualType\": Value Change" {
          selector: w340 -> [_ _ _ _ _ _ _ _ _ _ _ _ _ _ _ _ _ _ _ _ _ _ _ _ _ _ _ _ _ _ _ _ _ _ _ _ _ _ _ _ _ _ _ _ _ _ _ _ _ _ _ _ _ _ _ _ _ _ _ _ _ _ _ _ _ _ _ _ _ _ _ _ _ _ _ _ _ _ _ _ _ _ _ _ _ _ _ _ _ _ _ _ _ _ _ _ _ _ _ _ _ _ _ _ _ _ _ _ _ _ _ _ _ _ _]
          dyn-events: _ -> [_ _ _ _ _ _ _ _ _ _ _ _ _ _ _ _ _ _ _ _ _ _ _ _ _ _ _ _ _ _ _ _ _ _ _ _ _ _ _ _ _ _ _ _ _ _ _ _ _ _ _ _ _ _ _ _ _ _ _ _ _ _ _ _ _ _ _ _ _ _ _ _ _ _ _ _ _ _ _ _ _ _ _ _ _ _ _ _ _ _ _ _ _ _ _ _ _ _ _ _ _ _ _ _ _ _ _ _ _ _ _ _ _ _ _]
          timeout: _ -> [_ _ _ _ _ _ _ _ _ _ _ _ _ _ _ _ _ _ _ _ _ _ _ _ _ _ _ _ _ _ _ _ _ _ _ _ _ _ _ _ _ _ _ _ _ _ _ _ _ _ _ _ _ _ _ _ _ _ _ _ _ _ _ _ _ _ _ _ _ _ _ _ _ _ _ _ _ _ _ _ _ _ _ _ _ _ _ _ _ _ _ _ _ _ _ _ _ _ _ _ _ _ _ _ _ _ _ _ _ _ _ _ _ _ _]
          tunnel: [FALSE ("NewVal") FALSE ("NewVal") FALSE ("NewVal") w365 FALSE ("NewVal") FALSE ("NewVal") FALSE ("NewVal") FALSE ("NewVal") FALSE ("NewVal") FALSE ("NewVal") FALSE ("NewVal") FALSE ("NewVal") FALSE ("NewVal") FALSE ("NewVal") FALSE ("NewVal") FALSE ("NewVal") FALSE ("NewVal") FALSE ("NewVal") FALSE ("NewVal") FALSE ("NewVal") FALSE ("NewVal") FALSE ("NewVal") FALSE ("NewVal") FALSE ("NewVal") FALSE ("NewVal") FALSE ("NewVal") FALSE ("NewVal") FALSE ("NewVal") FALSE ("NewVal") FALSE ("NewVal") FALSE ("NewVal") FALSE ("NewVal") FALSE ("NewVal") FALSE ("NewVal") w1218 FALSE ("NewVal") FALSE ("NewVal") FALSE ("NewVal") FALSE ("NewVal") FALSE ("NewVal") FALSE ("NewVal") FALSE ("NewVal") FALSE ("NewVal") FALSE ("NewVal") FALSE ("NewVal") FALSE ("NewVal") FALSE ("NewVal") FALSE ("NewVal") FALSE ("NewVal") FALSE ("NewVal") FALSE ("NewVal") FALSE ("NewVal") FALSE ("NewVal") FALSE ("NewVal") FALSE ("NewVal") FALSE ("NewVal") FALSE ("NewVal") FALSE ("NewVal") FALSE ("NewVal") FALSE ("NewVal") FALSE ("NewVal") FALSE ("NewVal") FALSE ("NewVal") FALSE ("NewVal") FALSE ("NewVal") FALSE ("NewVal") FALSE ("NewVal") FALSE ("NewVal") FALSE ("NewVal") FALSE ("NewVal") FALSE ("NewVal") FALSE ("NewVal") FALSE ("NewVal") FALSE ("NewVal") FALSE ("NewVal") FALSE ("NewVal") FALSE ("NewVal") FALSE ("NewVal") FALSE ("NewVal") FALSE ("NewVal") FALSE ("NewVal") FALSE ("NewVal") FALSE ("NewVal") FALSE ("NewVal") FALSE ("NewVal") FALSE ("NewVal") FALSE ("NewVal") FALSE ("NewVal") FALSE ("NewVal") FALSE ("NewVal") FALSE ("NewVal") FALSE ("NewVal") FALSE ("NewVal") FALSE ("NewVal") FALSE ("NewVal") FALSE ("NewVal") FALSE ("NewVal") FALSE ("NewVal") FALSE ("NewVal") FALSE ("NewVal") FALSE ("NewVal") FALSE ("NewVal") FALSE ("NewVal") FALSE ("NewVal") FALSE ("NewVal") FALSE ("NewVal") FALSE ("NewVal") FALSE ("NewVal") FALSE ("NewVal") FALSE ("NewVal") FALSE ("NewVal") FALSE ("NewVal") FALSE ("NewVal") FALSE ("NewVal") FALSE ("NewVal")] -> w341
          event Timeout {
            n671 = event-data() -> ()  [unwired: 1 in, 2 out]
          }
          event "RecordSel": Value Change {
            n672 = event-data() -> ("NewVal"=w344:string)  [unwired: 1 in, 4 out]
            n673 = local read "DatabaseUDL"() -> (w347:path)
            n674 = call "FeedbackDecode_UpdateDatabase.vi"("RecordsSelection"=w344, "CallType"=enum16{"Initialize", "Save", "Load"}."Load", "DatabaseUDL"=w347) -> ("DatabaseOut"=w345:T12)  [unwired: 1 in, 2 out]
            n675 = local write "Database"(w345) -> ()
          }
          event "SendComment": Value Change {
            n676 = event-data() -> ("NewVal"=w349:bool)  [unwired: 1 in, 4 out]
            n677 = case shown="True" w349 {
              frame False {
              }
              frame True {
                n678 = stacked-sequence {
                  frame #0 {
                    n679 = local read "LoopCnt"() -> (w358:u64)
                    n680 = local read "NIPTime"() -> (w354:dbl)
                    n681 = local read "Comment"() -> (w361:string)
                    n682 = Format Into String(w358) -> (resulting string=w350:string)  [unwired: 3 in, 1 out]
                    n683 = call-poly "FeedbackDecode_VariablesToString.vi"("Format"="%0.0f", "ValueIn"=w354, "FieldName"="NIPTime" ("Key Word")) -> ("StringOut"=w351:string)  [unwired: 4 in]
                    n684 = Concatenate Strings("SendComment:SS.EventID=" ("string"), w350) -> (w357:string)
                    n685 = local read "EventParamsFID"() -> (w356:refnum<file>)
                    n686 = Concatenate Strings(w357, ";SS.Comment='" ("string"), w361, "';" ("string"), w351) -> (w355:string)
                    n687 = call "FeedbackDecode_WriteTextEOL.vi"("text"=w355, "refnum in"=w356) -> ()  [unwired: 8 in, 2 out]
                  }
                  frame #1 {
                    n688 = local write "SendComment"(FALSE ("SendComment")) -> ()
                    n689 = local write "Comment"("" ("Comment")) -> ()
                  }
                }
              }
            }
          }
          event Value Change {
            n690 = event-data() -> ("NewVal"=w366:bool)  [unwired: 1 in, 4 out]
            n691 = case shown="True" w366 {
              tunnel: [FALSE ("NewVal") FALSE ("NewVal")] -> w365
              frame False {
                n692 = local read "LoopCnt"() -> (w378:u64)
                n693 = local read "NIPTime"() -> (w371:dbl)
                n694 = Format Into String(w378) -> (resulting string=w367:string)  [unwired: 3 in, 1 out]
                n695 = call-poly "FeedbackDecode_VariablesToString.vi"("Format"="%0.0f", "ValueIn"=w371, "FieldName"="NIPTime" ("Key Word")) -> ("StringOut"=w368:string)  [unwired: 4 in]
                n696 = Concatenate Strings("StopTraining:SS.EventID=" ("string"), w367) -> (w377:string)
                n697 = local read "EventParamsFID"() -> (w375:refnum<file>)
                n698 = Concatenate Strings(w377, ";SS.AcqTraining=0;" ("EventStr"), w368) -> (w374:string)
                n699 = local read "DecodeClust"() -> (w386:T5)
                n700 = call "FeedbackDecode_WriteTextEOL.vi"("text"=w374, "refnum in"=w375) -> ()  [unwired: 8 in, 2 out]
                n701 = Bundle By Name(cluster=w386, "EventStr"=w374) -> (w373:T5)
                n702 = call "FeedbackDecode_MLComCtrl.vi"("DecodeClustIn"=w373, "Mode"=T19."SendEvent") -> ("DecodeClustOut"=w372:T5)  [unwired: 6 in, 3 out]
                n703 = Unbundle By Name(w372) -> ("CtrlButtons.StartTrials"=w383:bool)
                n704 = And(x=w383, y=FALSE) -> (x .and. y?=w381:bool)
                n705 = property on="StartTrials" class="Bool (strict)"("Value"=w381) -> (error out=w380:errorcluster)  [unwired: 2 in, 1 out]
                n706 = property on="ApplyBaseline" class="Bool (strict)"(error in=w380, "DisabledEnum"=T17."Enabled" ("Disabled")) -> ()  [unwired: 1 in, 2 out]
              }
              frame True {
                n707 = local read "NIPTime"() -> (w393:dbl)
                n708 = local read "LoopCnt"() -> (w402:u64)
                n709 = call-poly "FeedbackDecode_VariablesToString.vi"("Format"="%0.0f", "ValueIn"=w393, "FieldName"="NIPTime" ("Key Word")) -> ("StringOut"=w390:string)  [unwired: 4 in]
                n710 = Format Into String(w402) -> (resulting string=w389:string)  [unwired: 3 in, 1 out]
                n711 = local read "EventParamsFID"() -> (w399:refnum<file>)
                n712 = Concatenate Strings("StartTraining:SS.EventID=" ("string"), w389) -> (w401:string)
                n713 = Concatenate Strings(w401, ";SS.AcqTraining=1;" ("EventStr"), w390) -> (w398:string)
                n714 = local read "DecodeClust"() -> (w408:T5)
                n715 = call "FeedbackDecode_WriteTextEOL.vi"("text"=w398, "refnum in"=w399) -> ()  [unwired: 8 in, 2 out]
                n716 = Bundle By Name(cluster=w408, "EventStr"=w398) -> (w397:T5)
                n717 = call "FeedbackDecode_MLComCtrl.vi"("DecodeClustIn"=w397, "Mode"=T19."SendEvent") -> ("DecodeClustOut"=w396:T5)  [unwired: 6 in, 3 out]
                n718 = Unbundle By Name(w396) -> ("ReTrain"=w409:bool)
                n719 = case shown="True" w409 {
                  tunnel: [w412 w414] -> w395
                  frame False {
                    n720 = property on="KinSrc" class="Enum (strict)"("Val(Sgnl)"=enum16{"Off", "Training", "Decode", "COB"}."Training" ("Value (Signaling)")) -> (error out=w412:errorcluster)  [unwired: 2 in, 1 out]
                  }
                  frame True {
                    n721 = property on="KinSrc" class="Enum (strict)"("Val(Sgnl)"=enum16{"Off", "Training", "Decode", "COB"}."Decode" ("Value (Signaling)")) -> (error out=w414:errorcluster)  [unwired: 2 in, 1 out]
                  }
                }
                n722 = property on="TestType" class="Enum (strict)"(error in=w395, "Val(Sgnl)"=T23."MSMS" ("Value (Signaling)")) -> (error out=w394:errorcluster)  [unwired: 1 in, 1 out]
                n723 = property on="StartTrials" class="Bool (strict)"(error in=w394, "Val(Sgnl)"=TRUE ("Value (Signaling)")) -> (error out=w404:errorcluster)  [unwired: 1 in, 1 out]
                n724 = property on="ApplyBaseline" class="Bool (strict)"(error in=w404, "DisabledEnum"=T17."Disabled and Grayed Out" ("Disabled")) -> ()  [unwired: 1 in, 2 out]
              }
            }
          }
          event Value Change {
            n725 = event-data() -> ("NewVal"=w416:bool)  [unwired: 1 in, 5 out]
            n726 = case shown="True" w416 {
              frame False {
                n727 = local read "LoopCnt"() -> (w427:u64)
                n728 = local read "NIPTime"() -> (w421:dbl)
                n729 = Format Into String(w427) -> (resulting string=w417:string)  [unwired: 3 in, 1 out]
                n730 = call-poly "FeedbackDecode_VariablesToString.vi"("Format"="%0.0f", "ValueIn"=w421, "FieldName"="NIPTime" ("Key Word")) -> ("StringOut"=w418:string)  [unwired: 4 in]
                n731 = Concatenate Strings("StopAcqBaseline:SS.EventID=" ("string"), w417) -> (w426:string)
                n732 = local read "EventParamsFID"() -> (w424:refnum<file>)
                n733 = local read "DecodeClust"() -> (w430:T5)
                n734 = Concatenate Strings(w426, ";SS.AcqBaseline=0;" ("EventStr"), w418) -> (w423:string)
                n735 = call "FeedbackDecode_WriteTextEOL.vi"("text"=w423, "refnum in"=w424) -> ()  [unwired: 8 in, 2 out]
                n736 = Bundle By Name(cluster=w430, "EventStr"=w423) -> (w422:T5)
                n737 = call "FeedbackDecode_MLComCtrl.vi"("DecodeClustIn"=w422, "Mode"=T19."SendEvent") -> ()  [unwired: 6 in, 4 out]
              }
              frame True {
                n738 = local read "LoopCnt"() -> (w441:u64)
                n739 = local read "NIPTime"() -> (w435:dbl)
                n740 = Format Into String(w441) -> (resulting string=w431:string)  [unwired: 3 in, 1 out]
                n741 = Concatenate Strings("StartAcqBaseline:SS.EventID=" ("string"), w431) -> (w440:string)
                n742 = call-poly "FeedbackDecode_VariablesToString.vi"("Format"="%0.0f", "ValueIn"=w435, "FieldName"="NIPTime" ("Key Word")) -> ("StringOut"=w432:string)  [unwired: 4 in]
                n743 = local read "EventParamsFID"() -> (w438:refnum<file>)
                n744 = local read "DecodeClust"() -> (w444:T5)
                n745 = Concatenate Strings(w440, ";SS.AcqBaseline=1;" ("EventStr"), w432) -> (w437:string)
                n746 = call "FeedbackDecode_WriteTextEOL.vi"("text"=w437, "refnum in"=w438) -> ()  [unwired: 8 in, 2 out]
                n747 = Bundle By Name(cluster=w444, "EventStr"=w437) -> (w436:T5)
                n748 = call "FeedbackDecode_MLComCtrl.vi"("DecodeClustIn"=w436, "Mode"=T19."SendEvent") -> ()  [unwired: 6 in, 4 out]
              }
            }
          }
          event "Exclude SE": Value Change {
            n749 = event-data() -> ("NewVal"=w446:bool)  [unwired: 1 in, 5 out]
            n750 = case shown="True" w446 {
              frame False {
                n751 = local read "LoopCnt"() -> (w457:u64)
                n752 = local read "NIPTime"() -> (w451:dbl)
                n753 = Format Into String(w457) -> (resulting string=w447:string)  [unwired: 3 in, 1 out]
                n754 = call-poly "FeedbackDecode_VariablesToString.vi"("Format"="%0.0f", "ValueIn"=w451, "FieldName"="NIPTime" ("Key Word")) -> ("StringOut"=w448:string)  [unwired: 4 in]
                n755 = Concatenate Strings("ExcludeSE:SS.EventID=" ("string"), w447) -> (w456:string)
                n756 = local read "EventParamsFID"() -> (w454:refnum<file>)
                n757 = local read "DecodeClust"() -> (w460:T5)
